vi "debug_array_crash.vi"() -> ()   [LabVIEW 2015]
panel:
  out "subarray":dbl[](array[numeric])
  out "2-D Array of Real 2":dbl[][](array[numeric])
  out "2-D Array of Real":dbl[][](array[numeric])
  out "labviewX":dbl[](array[numeric])
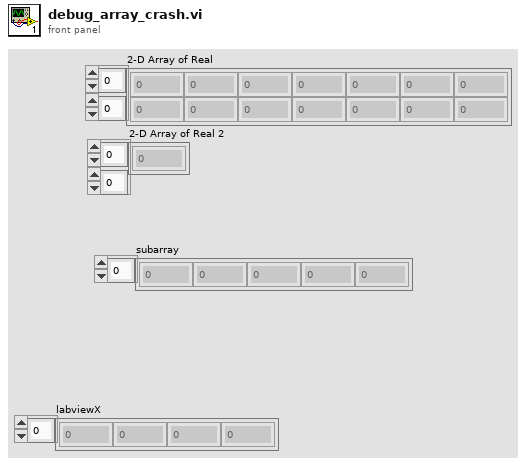
[diagram p1: front panel]
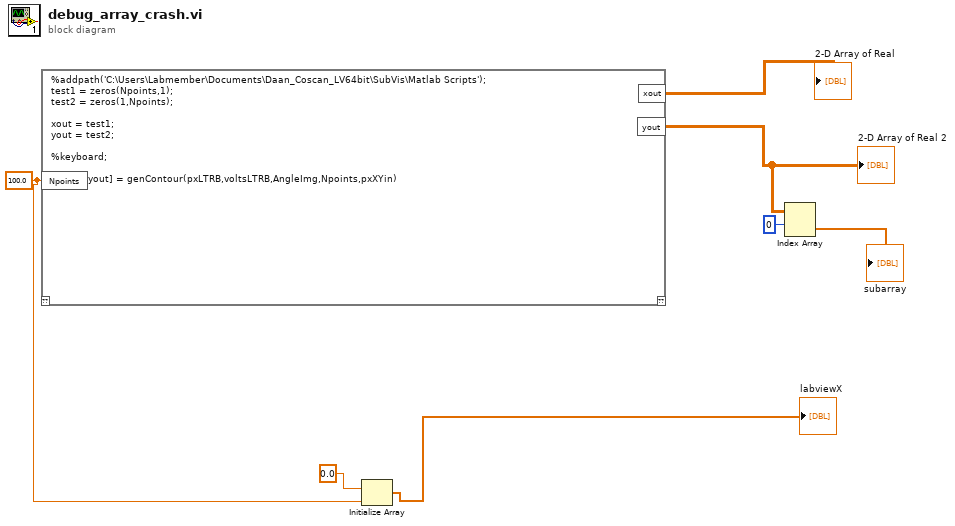
[diagram p0: block diagram]
diagram:
  w4 = 100.0 ("Real")
  n1 = script code="%addpath('C:\\Users\\Labmember\\Documents\\Daan_Coscan_LV64bit\\SubVis\\Matlab Scripts');\ntest1 = zeros(Npoints,1);\ntest2 = zeros(1,Npoints);\n\nxout = test1;\nyout = test2;\n\n%keyboard;\n\n%[xout yout] = genContour(pxLTRB,voltsLTRB,AngleImg,Npoints,pxXYin)"("Npoints"=w4) -> ("xout"=→"2-D Array of Real":dbl[][], "yout"=w3:dbl[][])  [unwired: 1 in, 1 out]
  "2-D Array of Real 2" <- w3
  n2 = Initialize Array(0.0 ("P"), w4) -> (→"labviewX":dbl[])
  n3 = Index Array(array=w3, index (row)=0) -> (element=→"subarray":dbl[])  [unwired: 1 in]
